vi "JKISM++ Generate User Global Log.vi"(6 "From Who":string, 7 "ModuleName":string, 8 "Error in":errorcluster caption="Error in (no error)", 10 "Arguments":string, 11 "Log":string) -> (0 "error out":errorcluster)   [LabVIEW 2014, in "JKI State Machine++.lvlib"]
uses:
  JKI State Machine++.lvlib
  _Support/Typedef/_JKISM_GlobalLog_MSG.ctl
  _Support/Typedef/_JKISM_GlobalLog_MSG_TYPE.ctl
  _Support/GlobalEvent/FGV-GlobalEventRef.vi
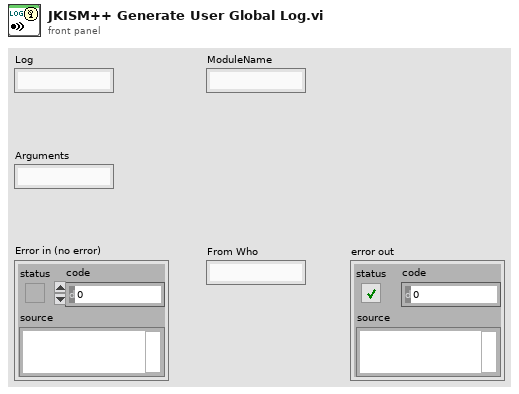
[diagram p1: front panel]
types:
  T1 = typedef "JKI State Machine++.lvlib/_JKISM_GlobalLog_MSG_TYPE.ctl" = enum16{"User Log", "State Change", "Status Change", "Interrupt Change", "Register", "Unregister"}
  T2 = typedef "JKI State Machine++.lvlib/_JKISM_GlobalLog_MSG.ctl" = cluster{"Name(\"\" to use uuid)":string, "Current State":string, "Arguments":string, "Argument - State":string, "From Who":string, "Complete(T)/Start(F)":bool, "Type":T1}
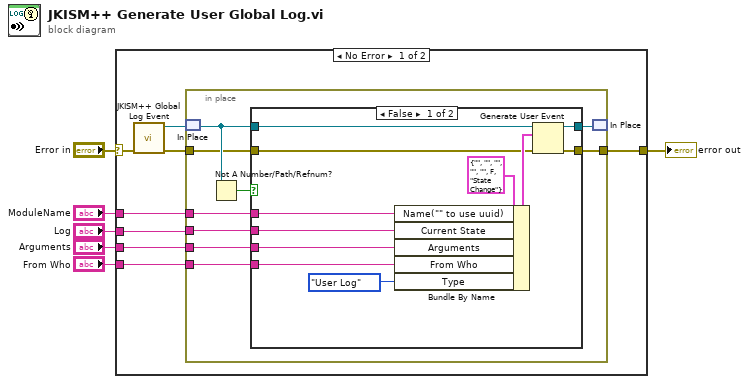
[diagram p0: block diagram]
diagram:
  n1 = case shown="No Error" "Error in" {
    selector: "Error in" -> [w11 w37]
    tunnel: [w12 w37] -> w6
    tunnel: "From Who" -> [w10 _]
    tunnel: "ModuleName" -> [w9 _]
    tunnel: "Log" -> [w8 _]
    tunnel: "Arguments" -> [w7 _]
    frame No Error {
      n2 = call "JKISM++ Global Log Event.vi"("Error in"=w11) -> ("Error out"=w13:errorcluster, "JKISM Global Log Event"=w14:refnum<user-event>)  [unwired: 9 in]
      n3 = in-place {
        in-place-border: w9 -> [w20]
        in-place-border: w8 -> [w19]
        in-place-border: w7 -> [w18]
        in-place-border: w13 -> [w17]
        in-place-border: [w16] -> w12
        in-place-border: w10 -> [w15]
        n4 = in-place-match #1(w14) -> (w22:refnum<user-event>)
        n5 = Not A Number/Path/Refnum?(number/path/refnum=w22) -> (NaN/Path/Refnum?=w23:bool)
        n6 = case shown="False" w23 {
          tunnel: w22 -> [w34 w36]
          tunnel: w20 -> [w31 _]
          tunnel: [w30 w36] -> w21
          tunnel: w19 -> [w29 _]
          tunnel: w18 -> [w28 _]
          tunnel: w17 -> [w27 w35]
          tunnel: [w26 w35] -> w16
          tunnel: w15 -> [w24 _]
          frame False {
            n7 = Bundle By Name(cluster=T2 {"Name(\"\" to use uuid)"="", "Current State"="", "Arguments"="", "Argument - State"="", "From Who"="", "Complete(T)/Start(F)"=FALSE, "Type"=enum."State Change"} ("event data"), "Name(\"\" to use uuid)"=w31, "Current State"=w29, "Arguments"=w28, "From Who"=w24, "Type"=_JKISM_GlobalLog_MSG_TYPE."User Log") -> (w32:T2)
            n8 = Generate User Event(user event=w34, event data cluster=w32, error in=w27) -> (user event out=w30:refnum<user-event>, error out=w26:errorcluster)  [unwired: 1 in]
          }
          frame True {
          }
        }
        n9 = in-place-match #1(w21) -> ()  [unwired: 1 out]
      }
    }
    frame Error {
    }
  }
  "error out" <- w6
